vi "evaluateBooleanParsingUppercase.vi"(8 "error in (no error)":errorcluster, 11 "TestCase in":refnum<class "EasyXML_XML_Subset_Evaluations.lvclass">) -> (0 "error out":errorcluster, 3 "TestCase out":refnum<class "EasyXML_XML_Subset_Evaluations.lvclass">)   [LabVIEW 2013, in "EasyXML_XML_Subset_Evaluations.lvclass"]
doc: "Verify that error in is not overwritten"
uses:
  EasyXML_XML_Subset_Evaluations.lvclass
panel:
  out "Produced Data":variant
  out "Expected Data":variant
  out "XML String":string
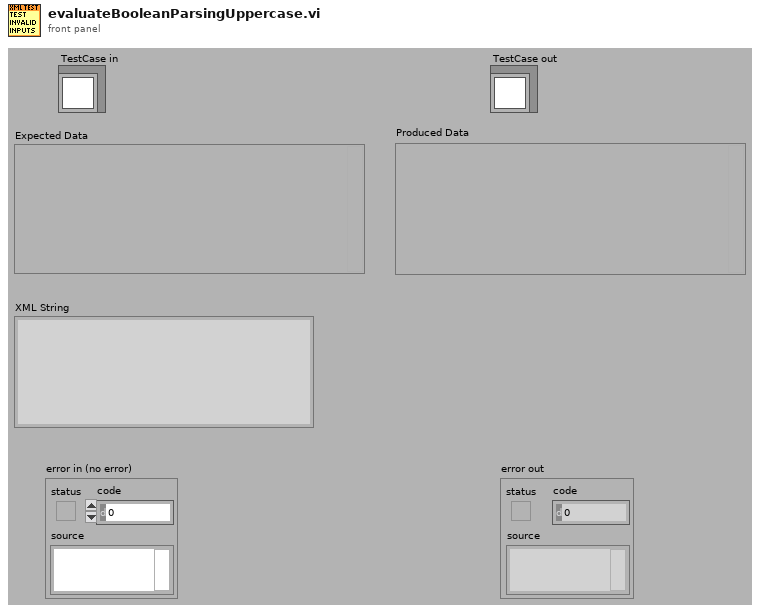
[diagram p1: front panel]
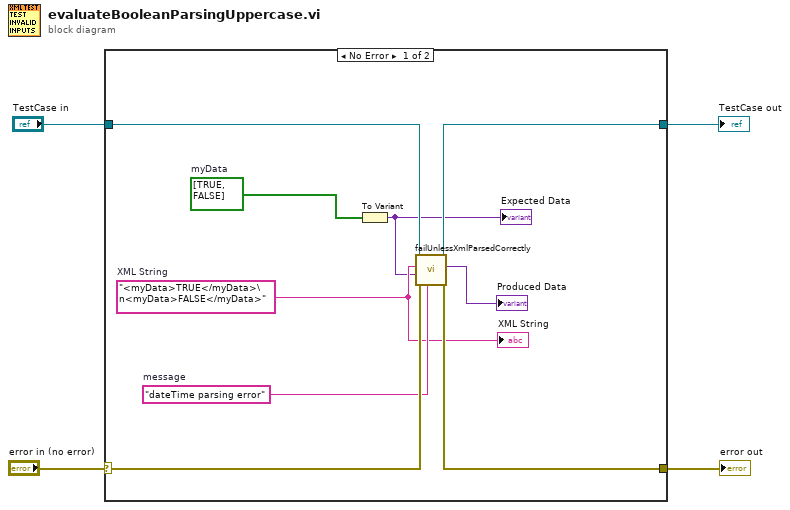
[diagram p0: block diagram]
diagram:
  n1 = case shown="No Error" "error in (no error)" {
    selector: "error in (no error)" -> [w12 w15]
    tunnel: [w11 w15] -> w2
    tunnel: [w10 w14] -> w1
    tunnel: "TestCase in" -> [w13 w14]
    frame No Error {
      w5 = bool[] [TRUE, FALSE]  # myData
      w8 = "<myData>TRUE</myData>\n<myData>FALSE</myData>"  # XML String
      w9 = "dateTime parsing error"  # message
      n2 = To Variant(anything=w5) -> (Variant=w7:variant)
      "Expected Data" <- w7
      n3 = call "failUnlessXmlParsedCorrectly.vi"("message (\"\")"=w9, "error in"=w12, "Expected Data"=w7, "XML String"=w8, "reference in"=w13) -> ("error out"=w11:errorcluster, "Produced Data"=→"Produced Data":variant, "reference in"=w10:refnum<class "EasyXML_XML_Subset_Evaluations.lvclass">)  [unwired: 4 in]
      "XML String" <- w8
    }
    frame Error {
    }
  }
  "error out" <- w2
  "TestCase out" <- w1
